vi "GetMap.vi"(8 "error in (no error)":errorcluster, 10 "size":i32, 11 "MsgPackDeserializer in":refnum<class "MsgPackDeserializer.lvclass">) -> (0 "error out":errorcluster, 2 "Variant":variant, 3 "MsgPackDeserializer out":refnum<class "MsgPackDeserializer.lvclass">)   [LabVIEW 2015, in "MsgPackDeserializer.lvclass"]
uses:
  MsgPackDeserializer.lvclass
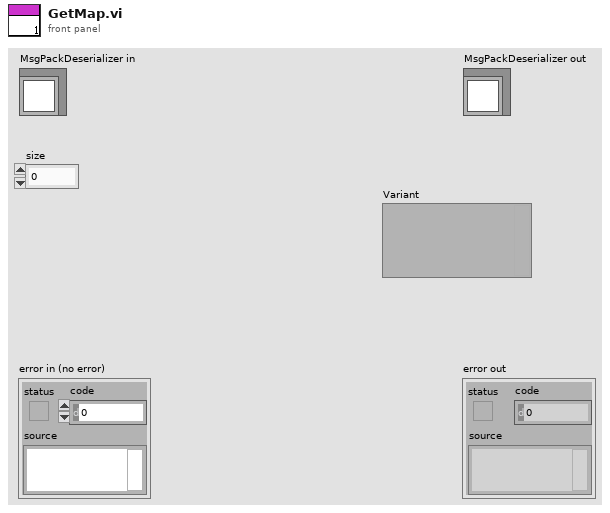
[diagram p1: front panel]
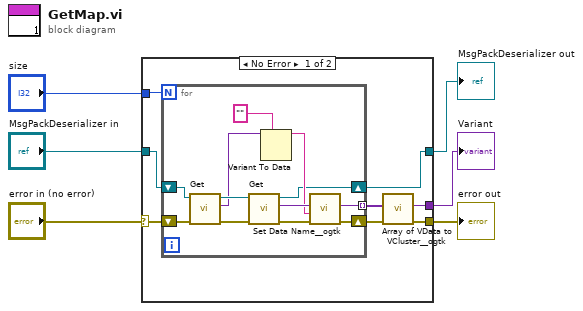
[diagram p0: block diagram]
diagram:
  n1 = case shown="No Error" "error in (no error)" {
    selector: "error in (no error)" -> [w10 w28]
    tunnel: [w9 w28] -> w5
    tunnel: [w7 w27] -> w3
    tunnel: "MsgPackDeserializer in" -> [w12 w27]
    tunnel: [w11 _] -> w2
    tunnel: "size" -> [w8 _]
    frame No Error {
      n2 = for {
        N: w8 -> [_]
        shift-right: [w26] -> w13
        shift-left: w10 -> [w18]
        tunnel: [w25] -> w14 mode=indexing
        shift-right: [w15] -> w7
        shift-left: w12 -> [w19]
        n3 = call "Get.vi"("error in (no error)"=w18, "MsgPackDeserializer in"=w19) -> ("error out"=w17:errorcluster, "Variant"=w23:variant, "MsgPackDeserializer out"=w24:refnum<class "MsgPackDeserializer.lvclass">)  [unwired: 7 in]
        n4 = call "Get.vi"("error in (no error)"=w17, "MsgPackDeserializer in"=w24) -> ("error out"=w16:errorcluster, "Variant"=w21:variant, "MsgPackDeserializer out"=w15:refnum<class "MsgPackDeserializer.lvclass">)  [unwired: 7 in]
        n5 = Variant To Data(type="" ("Data Name"), Variant=w23) -> (data=w20:string)  [unwired: 1 in, 1 out]
        n6 = call <userlib>:"Set Data Name__ogtk.vi"("error in (no error)"=w16, "Data Name"=w20, "Data"=w21) -> ("error out"=w26:errorcluster, "Renamed Data"=w25:variant)  [unwired: 7 in]
      }
      n7 = call <userlib>:"Array of VData to VCluster__ogtk.vi"("error in (no error)"=w13, "Array"=w14) -> ("error out"=w9:errorcluster, "VCluster"=w11:variant)  [unwired: 8 in]
    }
    frame Error {
    }
  }
  "error out" <- w5
  "MsgPackDeserializer out" <- w3
  "Variant" <- w2
